vi "Flush.vi"(8 "error in (no error)":errorcluster, 11 "VISA resource name":refnum<visa-resource-name>) -> (0 "error out":errorcluster, 3 "VISA resource name out":refnum<visa-resource-name>)   [LabVIEW 2009, in "Digikrom DK24x.lvlib"]
doc: "Flushes all buffers associated with VISA resource."
uses:
  Digikrom DK24x.lvlib
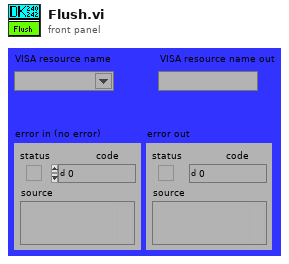
[diagram p1: front panel]
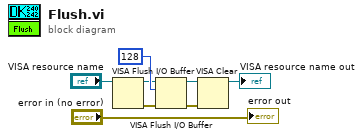
[diagram p0: block diagram]
diagram:
  n1 = VISA Flush I/O Buffer(VISA resource name="VISA resource name") -> (VISA resource name out=w7:refnum<visa-resource-name>, error out=w6:errorcluster)  [unwired: 2 in]
  n2 = VISA Flush I/O Buffer(VISA resource name=w7, mask (16)=128, error in (no error)=w6) -> (VISA resource name out=w2:refnum<visa-resource-name>, error out=w3:errorcluster)
  n3 = VISA Clear(VISA resource name=w2, error in (no error)=w3) -> (VISA resource name out=→"VISA resource name out":refnum<visa-resource-name>)  [unwired: 1 out]
  "error out" <- "error in (no error)"
